vi "FilterLittle.vi"(10 "Little Boat Queues":T2, 11 "NotifierReff":T1) -> ()   [LabVIEW 2013]
uses:
  Data/TypeDefs/UTM Location.ctl
  Data/TypeDefs/Notifiers.ctl
  Data/TypeDefs/Sail Set Suggestions.ctl
  Data/TypeDefs/Rudder Set Suggestions.ctl
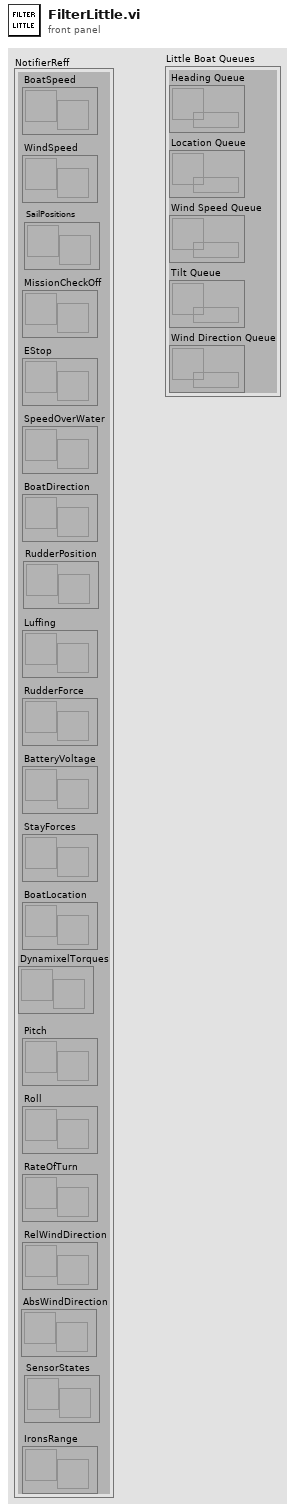
[diagram p1: front panel]
types:
  T1 = typedef "Notifiers.ctl" = cluster{"BoatSpeed":refnum<notifier>, "WindSpeed":refnum<notifier>, "MissionCheckOff":refnum<notifier>, "EStop":refnum<notifier>, "SpeedOverWater":refnum<notifier>, "BoatDirection":refnum<notifier>, "Luffing":refnum<notifier>, "RudderForce":refnum<notifier>, "BatteryVoltage":refnum<notifier>, "StayForces":refnum<notifier>, "BoatLocation":refnum<notifier>, "Pitch":refnum<notifier>, "Roll":refnum<notifier>, "RateOfTurn":refnum<notifier>, "RelWindDirection":refnum<notifier>, "SailPositions":refnum<notifier>, "RudderPosition":refnum<notifier>, "IronsRange":refnum<notifier>, "AbsWindDirection":refnum<notifier>, "DynamixelTorques":refnum<notifier>, "SensorStates":refnum<notifier>}
  T2 = cluster{"Heading Queue":refnum<queue>, "Location Queue":refnum<queue>, "Wind Speed Queue":refnum<queue>, "Tilt Queue":refnum<queue>, "Wind Direction Queue":refnum<queue>}
  T3 = typedef "UTM Location.ctl" = cluster{"UTM Zone":dbl, "Hemisphere":enum16{"North", "South"}, "East":dbl, "North":dbl}
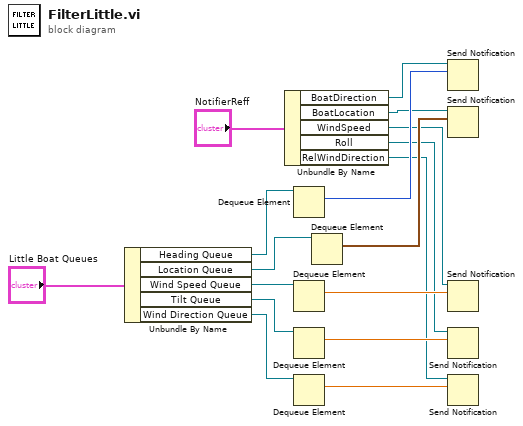
[diagram p0: block diagram]
diagram:
  n1 = Unbundle By Name("Little Boat Queues") -> ("Heading Queue"=w13:refnum<queue>, "Location Queue"=w10:refnum<queue>, "Wind Speed Queue"=w9:refnum<queue>, "Tilt Queue"=w8:refnum<queue>, "Wind Direction Queue"=w7:refnum<queue>)
  n2 = Unbundle By Name("NotifierReff") -> ("BoatDirection"=w15:refnum<notifier>, "BoatLocation"=w11:refnum<notifier>, "WindSpeed"=w3:refnum<notifier>, "Roll"=w2:refnum<notifier>, "RelWindDirection"=w1:refnum<notifier>)
  n3 = Dequeue Element(queue=w13) -> (element=w14:i32)  [unwired: 2 in, 3 out]
  n4 = Dequeue Element(queue=w9) -> (element=w6:dbl)  [unwired: 2 in, 3 out]
  n5 = Dequeue Element(queue=w8) -> (element=w5:dbl)  [unwired: 2 in, 3 out]
  n6 = Dequeue Element(queue=w7) -> (element=w4:dbl)  [unwired: 2 in, 3 out]
  n7 = Dequeue Element(queue=w10) -> (element=w12:T3)  [unwired: 2 in, 3 out]
  n8 = Send Notification(notification=w14, notifier=w15) -> ()  [unwired: 1 in, 2 out]
  n9 = Send Notification(notification=w12, notifier=w11) -> ()  [unwired: 1 in, 2 out]
  n10 = Send Notification(notification=w6, notifier=w3) -> ()  [unwired: 1 in, 2 out]
  n11 = Send Notification(notification=w5, notifier=w2) -> ()  [unwired: 1 in, 2 out]
  n12 = Send Notification(notification=w4, notifier=w1) -> ()  [unwired: 1 in, 2 out]
